vi "decodeStream.vi"(8 "error in (no error)":errorcluster, 9 "beginIndex":i32, 10 "binary stream":u8[](array[numeric]), 11 "tBSONRegEx in":refnum<class "tBSONRegEx.lvclass">) -> (0 "error out":errorcluster, 1 "endIndex":i32, 2 "binary stream out":u8[](array[numeric]), 3 "tBSONRegEx out":refnum<class "tBSONRegEx.lvclass">)   [LabVIEW 2013, in "BSON.lvlib" / "tBSONRegEx.lvclass"]
uses:
  tBSONRegEx.lvclass
  tBSONElement/tBSONElement.lvclass
  setRegularExpression.vi
  setOptionsString.vi
  BSON.lvlib
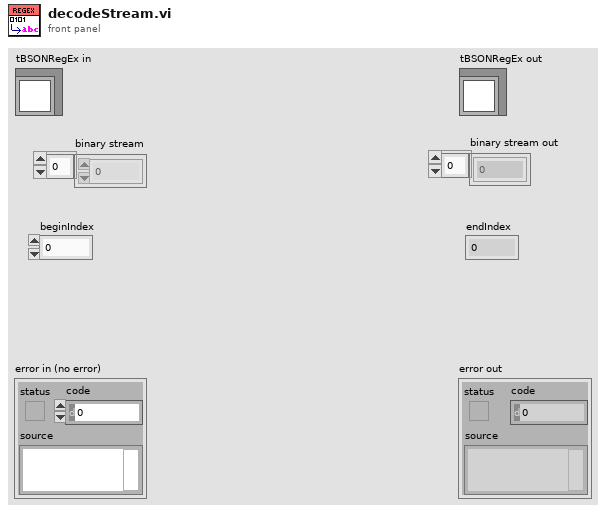
[diagram p1: front panel]
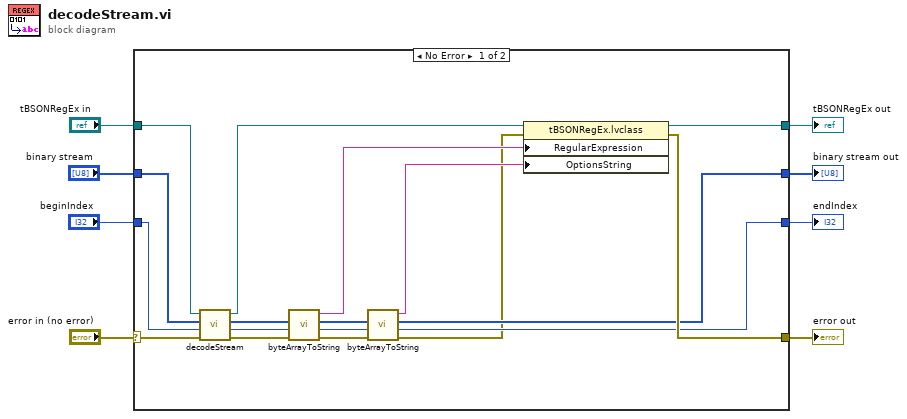
[diagram p0: block diagram]
diagram:
  n1 = case shown="No Error" "error in (no error)" {
    selector: "error in (no error)" -> [w26 w30]
    tunnel: [w13 w30] -> w1
    tunnel: "beginIndex" -> [w23 w29]
    tunnel: [w12 w29] -> w6
    tunnel: "binary stream" -> [w24 w28]
    tunnel: [w11 w28] -> w4
    tunnel: "tBSONRegEx in" -> [w25 w27]
    tunnel: [w15 w27] -> w2
    frame No Error {
      n2 = call-parent "decodeStream.vi"("error in (no error)"=w26, "beginIndex"=w23, "binary stream"=w24, "tBSONElement in"=w25) -> ("error out"=w22:errorcluster, "endIndex"=w20:i32, "binary stream out"=w21:u8[], "tBSONElement out"=w16:refnum<class "tBSONRegEx.lvclass">)  [unwired: 4 in]
      n3 = call "byteArrayToString.vi"("error in (no error)"=w22, "startIndex"=w20, "ByteArrayIn"=w21) -> ("error out"=w19:errorcluster, "endIndex"=w18:i32, "ByteArrayOut"=w17:u8[], "String"=w14:string)  [unwired: 5 in]
      n4 = call "byteArrayToString.vi"("error in (no error)"=w19, "startIndex"=w18, "ByteArrayIn"=w17) -> ("error out"=w9:errorcluster, "endIndex"=w12:i32, "ByteArrayOut"=w11:u8[], "String"=w10:string)  [unwired: 5 in]
      n5 = property class="tBSONRegEx.lvclass"(reference=w16, error in=w9, "RegularExpression"=w14, "OptionsString"=w10) -> (reference out=w15:refnum<class "tBSONRegEx.lvclass">, error out=w13:errorcluster)
    }
    frame Error {
    }
  }
  "error out" <- w1
  "tBSONRegEx out" <- w2
  "binary stream out" <- w4
  "endIndex" <- w6
